vi "Configure Measurement Characteristics (Eye Pattern).vi"(0 "VISA resource name":refnum<visa-resource-name>, 5 "Eye Window Start (40%)":i32, 7 "Eye Window Stop (60%)":i32, 9 "Start Measurement After (1 hit)":i32, 11 "error in (no error)":errorcluster) -> (4 "VISA resource name out":refnum<visa-resource-name>, 15 "error out":errorcluster)   [LabVIEW 2009, in "Agilent 8000 Series.lvlib"]
doc: "Configure Eye Pattern definition for color grade math operation. It configures Eye Window Start,Eye Window Stop and Eye Window Stopafter properties."
uses:
  Agilent 8000 Series.lvlib
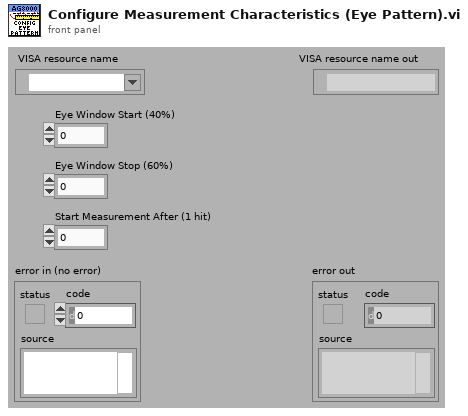
[diagram p1: front panel]
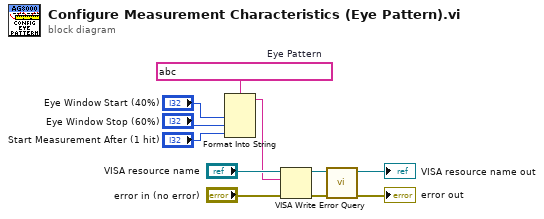
[diagram p0: block diagram]
diagram:
  w2 = string ?  # Eye Pattern
  n1 = Format Into String(format string=w2, "Eye Window Start (40%)", "Eye Window Stop (60%)", "Start Measurement After (1 hit)") -> (resulting string=w1:string)  [unwired: 2 in, 1 out]
  n2 = VISA Write(VISA resource name="VISA resource name", write buffer=w1, error in (no error)="error in (no error)") -> (VISA resource name out=w7:refnum<visa-resource-name>, error out=w6:errorcluster)  [unwired: 1 out]
  n3 = call "Error Query.vi"("error in (no error)"=w6, "VISA resource name"=w7) -> ("error out"=→"error out":errorcluster, "VISA resource name out"=→"VISA resource name out":refnum<visa-resource-name>)  [unwired: 6 in, 2 out]
